vi "Peak_selector_log (1).vi"(0 "Stasticl Parameters":T1, 1 "Array":ext[](array[numeric]), 2 "Array 2":i32[](array[numeric]), 4 "Hysteresis Spike":dbl, 5 "Length %":i32, 6 "MAX":dbl, 7 "Cut Amount":dbl, 8 "MIN":dbl=0.005, 9 "Step Height":i32=14) -> (3 "Boolean":bool)   [LabVIEW 2009]
uses:
  <vilib>/measure/mamon.llb/Trigger Detection for 1 Channel (obs).vi
  <vilib>/measure/NI_MAPro.lvlib
panel:
  out "total counts":i32
  out "Waveform Graph":i32[](graph)
  out "Boolean 2":bool
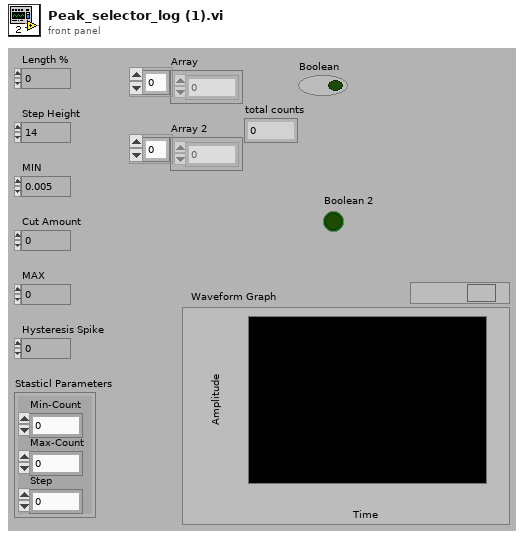
[diagram p1: front panel]
types:
  T1 = cluster{"Min-Count":sgl, "Max-Count":sgl, "Step":sgl}
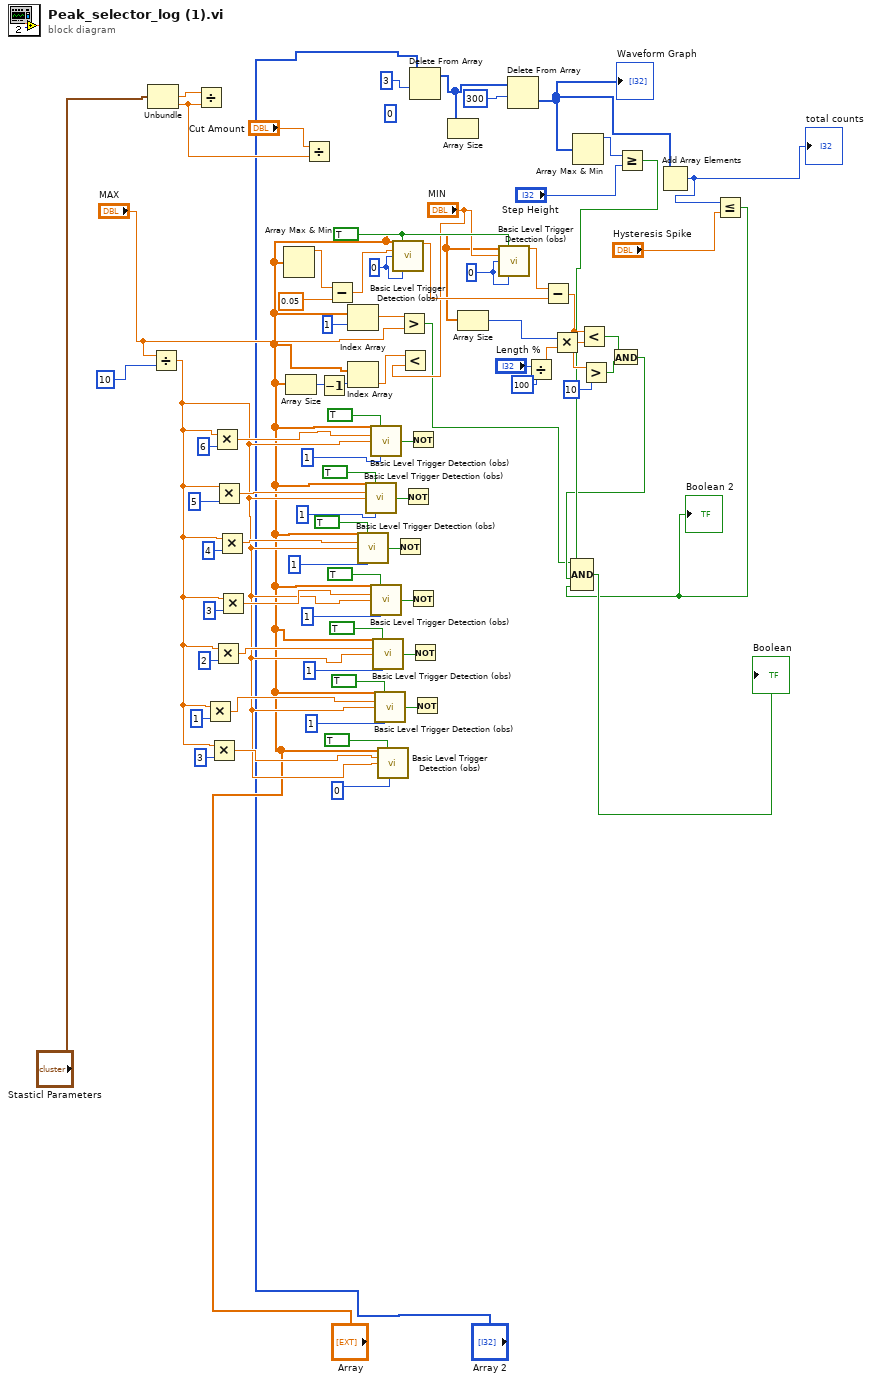
[diagram p0: block diagram]
diagram:
  (unwired) 0
  w45 = 0
  w44 = TRUE
  w43 = 0
  n1 = Unbundle("Stasticl Parameters") -> ("Max-Count"=w77:sgl, "Step"=w79:sgl)  [unwired: 1 out]
  n2 = Divide(x="MAX", y=10) -> (x/y=w13:dbl)
  n3 = Divide(x=w77, y=w79) -> ()  [unwired: 1 out]
  n4 = Multiply(x=w13, y=1) -> (x*y=w68:dbl)
  n5 = Multiply(x=w13, y=3) -> (x*y=w70:dbl)
  n6 = Multiply(x=w13, y=6) -> (x*y=w58:dbl)
  n7 = Multiply(x=w13, y=2) -> (x*y=w66:dbl)
  n8 = Multiply(x=w13, y=5) -> (x*y=w60:dbl)
  n9 = Multiply(x=w13, y=4) -> (x*y=w62:dbl)
  n10 = Multiply(x=w13, y=3) -> (x*y=w64:dbl)
  n11 = Array Max & Min(array="Array") -> (max value=w40:ext)  [unwired: 3 out]
  n12 = Array Size(array="Array") -> (size(s)=w27:i32)
  n13 = Divide(x="Cut Amount", y=w79) -> ()  [unwired: 1 out]
  n14 = Decrement(x=w27) -> (x-1=w19:i32)
  n15 = Subtract(x=w40, y=0.05) -> (x-y=w42:ext)
  n16 = Index Array(array="Array", index=1) -> (element=w17:ext)
  n17 = Index Array(array="Array", index=w19) -> (element=w18:ext)
  n18 = call-poly <vilib>:"Basic Level Trigger Detection (obs).vi"("signal in"="Array", "reset"=TRUE, "level"=w62, "hysteresis"=w13, "trigger slope"=1) -> ("trigger detected?"=w33:bool)  [unwired: 8 in, 2 out]
  n19 = call-poly <vilib>:"Basic Level Trigger Detection (obs).vi"("signal in"="Array", "reset"=TRUE, "level"=w60, "hysteresis"=w13, "trigger slope"=1) -> ("trigger detected?"=w35:bool)  [unwired: 8 in, 2 out]
  n20 = call-poly <vilib>:"Basic Level Trigger Detection (obs).vi"("signal in"="Array", "reset"=TRUE, "level"=w58, "hysteresis"=w13, "trigger slope"=1) -> ("trigger detected?"=w38:bool)  [unwired: 8 in, 2 out]
  n21 = call-poly <vilib>:"Basic Level Trigger Detection (obs).vi"("signal in"="Array", "reset"=TRUE, "level"=w64, "hysteresis"=w13, "trigger slope"=1) -> ("trigger detected?"=w30:bool)  [unwired: 8 in, 2 out]
  n22 = call-poly <vilib>:"Basic Level Trigger Detection (obs).vi"("signal in"="Array", "reset"=TRUE, "level"=w66, "hysteresis"=w13, "trigger slope"=1) -> ("trigger detected?"=w26:bool)  [unwired: 8 in, 2 out]
  n23 = call-poly <vilib>:"Basic Level Trigger Detection (obs).vi"("signal in"="Array", "reset"=TRUE, "level"=w68, "hysteresis"=w13, "trigger slope"=1) -> ("trigger detected?"=w22:bool)  [unwired: 8 in, 2 out]
  n24 = call-poly <vilib>:"Basic Level Trigger Detection (obs).vi"("signal in"="Array", "reset"=TRUE, "level"=w70, "hysteresis"=w13, "trigger slope"=0) -> ()  [unwired: 8 in, 3 out]
  n25 = call-poly <vilib>:"Basic Level Trigger Detection (obs).vi"("signal in"="Array", "reset"=w44, "level"=w42, "hysteresis"=w43, "trigger slope"=w43) -> ("trigger location"=w52:dbl)  [unwired: 8 in, 2 out]
  n26 = Not(x=w33) -> ()  [unwired: 1 out]
  n27 = Greater?(x=w17, y="MAX") -> (0:w6:bool)
  n28 = Less?(x=w18, y="MIN") -> ()  [unwired: 1 out]
  n29 = Not(x=w35) -> ()  [unwired: 1 out]
  n30 = Not(x=w38) -> ()  [unwired: 1 out]
  n31 = Not(x=w30) -> ()  [unwired: 1 out]
  n32 = Delete From Array(array="Array 2", length=3) -> (array with subset deleted=w9:i32[])  [unwired: 1 in, 1 out]
  n33 = Not(x=w26) -> ()  [unwired: 1 out]
  n34 = Not(x=w22) -> ()  [unwired: 1 out]
  n35 = Array Size(array=w9) -> ()  [unwired: 1 out]
  n36 = Array Size(array="Array") -> (size(s)=w71:i32)
  n37 = call-poly <vilib>:"Basic Level Trigger Detection (obs).vi"("signal in"="Array", "reset"=w44, "level"="MIN", "hysteresis"=w45, "trigger slope"=w45) -> ("trigger location"=w46:dbl)  [unwired: 8 in, 2 out]
  n38 = Delete From Array(array=w9, length=300) -> (deleted portion=w2:i32[])  [unwired: 1 in, 1 out]
  "Waveform Graph" <- w2
  n39 = Divide(x="Length %", y=100) -> (x/y=w74:dbl)
  n40 = Subtract(x=w46, y=w52) -> (x-y=w47:dbl)
  n41 = Multiply(x=w71, y=w74) -> (x*y=w72:dbl)
  n42 = Array Max & Min(array=w2) -> (max value=w53:i32)  [unwired: 3 out]
  n43 = Less?(x=w47, y=w72) -> (x < y?=w49:bool)
  n44 = Greater?(x=w47, y=10) -> (0:w50:bool)
  n45 = And(x=w49, y=w50) -> (x .and. y?=w7:bool)
  n46 = Greater Or Equal?(x=w53, y="Step Height") -> (x >= y?=w10:bool)
  n47 = Add Array Elements(numeric array=w2) -> (sum=w4:i32)
  "total counts" <- w4
  n48 = Less Or Equal?(x=w4, y="Hysteresis Spike") -> (x <= y?=w1:bool)
  "Boolean 2" <- w1
  n49 = Compound Arithmetic op=AND(w6, w10, w7, w1) -> (→"Boolean":bool)
